vi "GetValueFromModelFile.vi"(8 "error in (no error)":errorcluster caption="에러 입력(에러 없음)", 11 "init 파일 경로":string) -> (3 "출력 클러스터":T1)   [LabVIEW 2018]
uses:
  <vilib>/Utility/config.llb/NI_LVConfig.lvlib
  <vilib>/Utility/config.llb/Read Key (String).vi
  ModelFileData.ctl
  <vilib>/Utility/config.llb/Read Key (Double).vi
  <vilib>/Utility/config.llb/Read Key (U32).vi
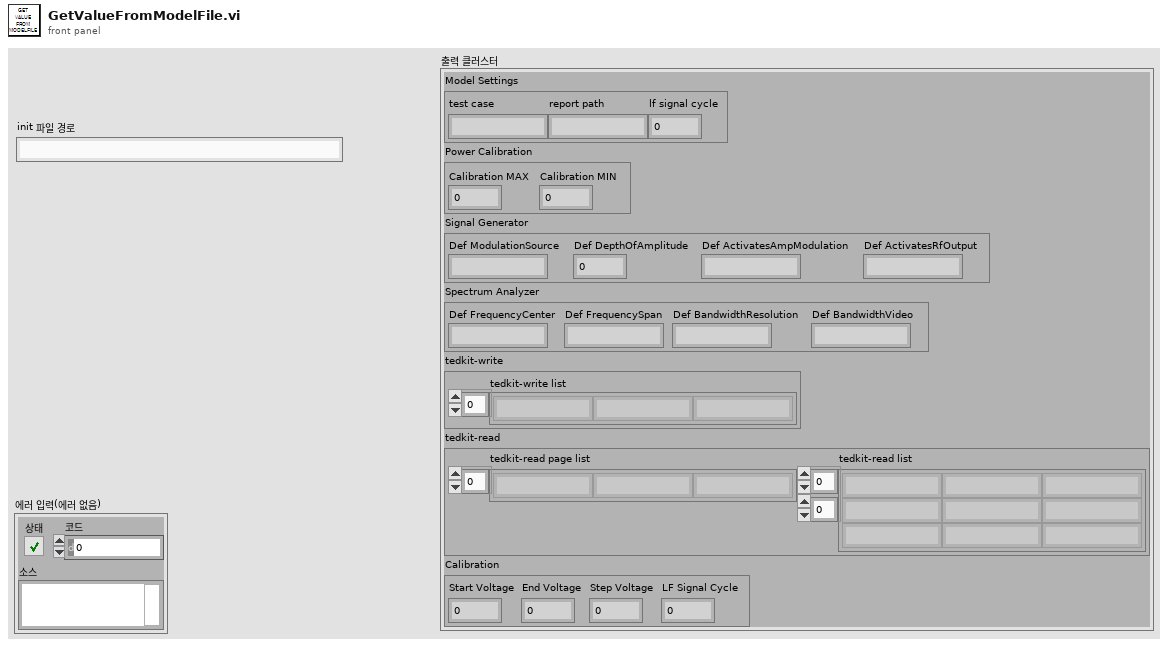
[diagram p1: front panel]
types:
  T1 = typedef "ModelFileData.ctl" = cluster{"Model Settings":cluster{"test case":string, "report path":string, "lf signal cycle":u16}, "Power Calibration":cluster{"Calibration MAX":dbl, "Calibration MIN":dbl}, "Signal Generator":cluster{"Def ModulationSource":string, "Def DepthOfAmplitude":dbl, "Def ActivatesAmpModulation":string, "Def ActivatesRfOutput":string}, "Spectrum Analyzer":cluster{"Def FrequencyCenter":string, "Def FrequencySpan":string, "Def BandwidthResolution":string, "Def BandwidthVideo":string}, "tedkit-write":cluster{"tedkit-write list":string[]}, "tedkit-read":cluster{"tedkit-read page list":string[], "tedkit-read list":string[][]}, "Calibration":cluster{"Start Voltage":dbl, "End Voltage":dbl, "Step Voltage":dbl, "LF Signal Cycle":u16}}
  T2 = typedef "NI_LVConfig.lvlib/Config Data RefNum.ctl" = refnum<k1>
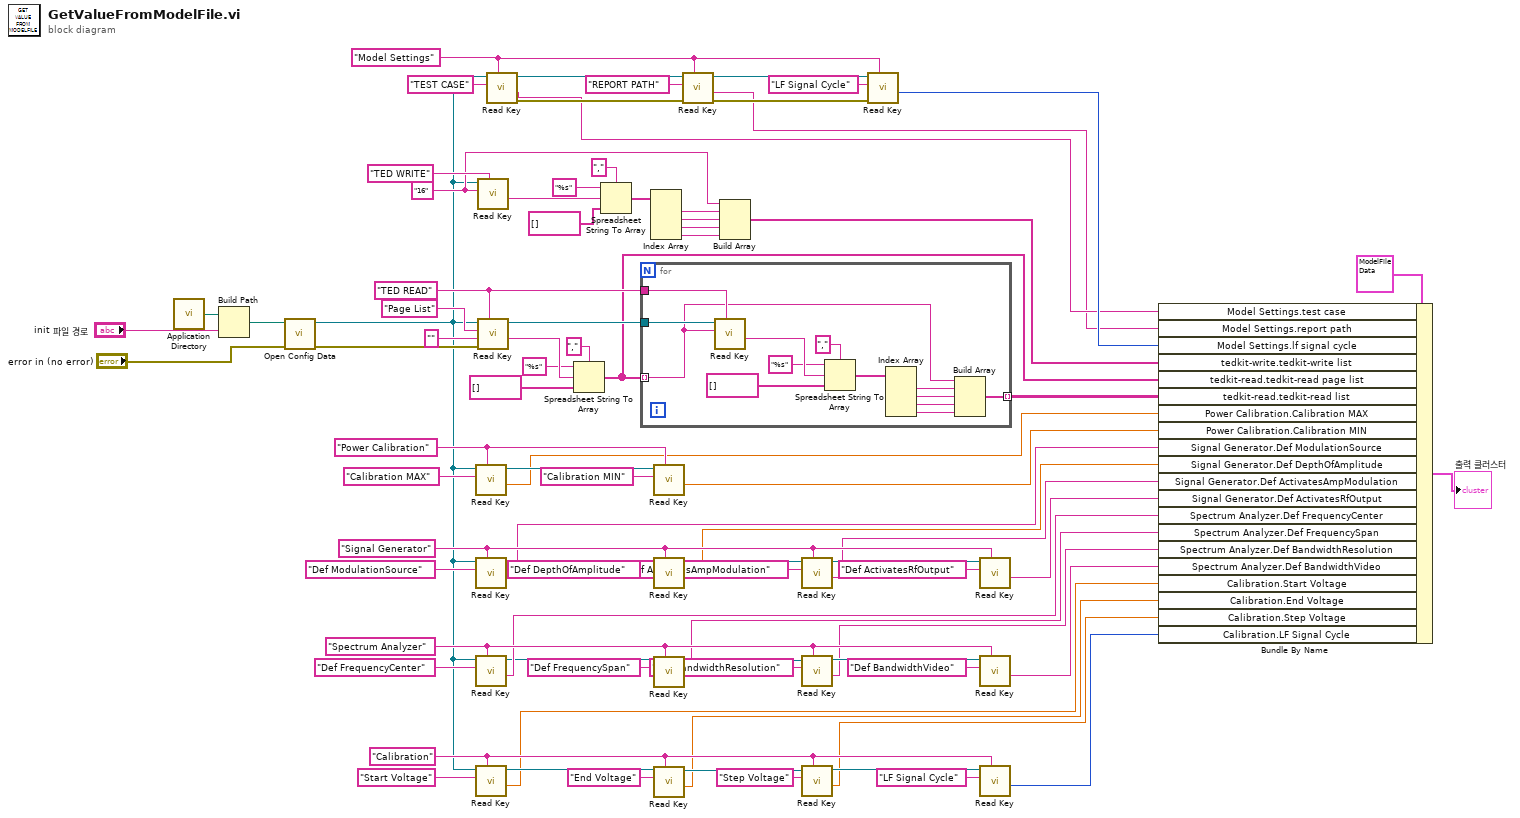
[diagram p0: block diagram]
diagram:
  w5 = "Model Settings" ("section")
  w22 = "Calibration" ("section")
  w33 = "Spectrum Analyzer" ("section")
  w46 = "Signal Generator" ("section")
  w25 = "16" ("key")
  w69 = "Power Calibration" ("section")
  w71 = "TED READ" ("section")
  n1 = call <vilib>:"Application Directory.vi"() -> ("Application Directory"=w83:path)
  n2 = Build Path(base path=w83, name or relative path="init 파일 경로") -> (appended path=w82:path)
  n3 = call <vilib>:"Open Config Data.vi"("error in (no error)"="error in (no error)", "configuration file path"=w82) -> ("error out"=w77:errorcluster, "refnum"=w12:T2)  [unwired: 7 in, 1 out]
  n4 = call-poly <vilib>:"Read Key.vi"("section"=w69, "key"="Calibration MAX", "refnum"=w12) -> ("value"=w63:dbl, "refnum out"=w70:T2)  [unwired: 5 in, 2 out]
  n5 = call-poly <vilib>:"Read Key.vi"("section"=w46, "key"="Def ModulationSource", "refnum"=w12) -> ("value"=w45:string, "refnum out"=w43:T2)  [unwired: 5 in, 2 out]
  n6 = call-poly <vilib>:"Read Key.vi"("section"=w33, "key"="Def FrequencyCenter", "refnum"=w12) -> ("value"=w32:string, "refnum out"=w27:T2)  [unwired: 5 in, 2 out]
  n7 = call-poly <vilib>:"Read Key.vi"("section"=w22, "key"="Start Voltage", "refnum"=w12) -> ("value"=w16:dbl, "refnum out"=w23:T2)  [unwired: 5 in, 2 out]
  n8 = call-poly <vilib>:"Read Key.vi"("section"="TED WRITE", "key"=w25, "refnum"=w12) -> ("value"=w59:string)  [unwired: 5 in, 3 out]
  n9 = call-poly <vilib>:"Read Key.vi"("section"=w71, "error in (no error)"=w77, "default value"="", "key"="Page List", "refnum"=w12) -> ("value"=w76:string, "refnum out"=w72:T2)  [unwired: 3 in, 2 out]
  n10 = call-poly <vilib>:"Read Key.vi"("section"=w5, "key"="TEST CASE", "refnum"=w12) -> ("error out"=w10:errorcluster, "value"=w2:string, "refnum out"=w9:T2)  [unwired: 5 in, 1 out]
  n11 = Spreadsheet String To Array(delimiter (Tab)="," ("구분 문자 (탭)"), format string="%s" ("포맷 문자열"), spreadsheet string=w76, array type (2D Dbl)=string[] [] ("배열 타입(2D Dbl)")) -> (array=w65:string[])
  n12 = Spreadsheet String To Array(delimiter (Tab)="," ("구분 문자 (탭)"), format string="%s" ("포맷 문자열"), spreadsheet string=w59, array type (2D Dbl)=string[] [] ("배열 타입(2D Dbl)")) -> (array=w57:string[])
  n13 = for {
    tunnel: w72 -> [w95]
    tunnel: w65 -> [w89] mode=indexing
    tunnel: w71 -> [w96]
    tunnel: [w84] -> w64 mode=indexing
    n14 = call-poly <vilib>:"Read Key.vi"("section"=w96, "key"=w89, "refnum"=w95) -> ("value"=w92:string)  [unwired: 5 in, 3 out]
    n15 = Spreadsheet String To Array(delimiter (Tab)="," ("구분 문자 (탭)"), format string="%s" ("포맷 문자열"), spreadsheet string=w92, array type (2D Dbl)=string[] [] ("배열 타입(2D Dbl)")) -> (array=w90:string[])
    n16 = Index Array(array=w90) -> (element #1=w88:string, element #2=w87:string, element #3=w86:string, element #4=w85:string)  [unwired: 4 in]
    n17 = Build Array(w89, w88, w87, w86, w85) -> (w84:string[])
  }
  n18 = Index Array(array=w57) -> (element #1=w56:string, element #2=w55:string, element #3=w54:string, element #4=w53:string)  [unwired: 4 in]
  n19 = call-poly <vilib>:"Read Key.vi"("section"=w69, "key"="Calibration MIN", "refnum"=w70) -> ("value"=w62:dbl)  [unwired: 5 in, 3 out]
  n20 = call-poly <vilib>:"Read Key.vi"("section"=w46, "key"="Def DepthOfAmplitude", "refnum"=w43) -> ("value"=w44:dbl, "refnum out"=w42:T2)  [unwired: 5 in, 2 out]
  n21 = call-poly <vilib>:"Read Key.vi"("section"=w33, "key"="Def FrequencySpan", "refnum"=w27) -> ("value"=w31:string, "refnum out"=w26:T2)  [unwired: 5 in, 2 out]
  n22 = call-poly <vilib>:"Read Key.vi"("section"=w22, "key"="End Voltage", "refnum"=w23) -> ("value"=w15:dbl, "refnum out"=w24:T2)  [unwired: 5 in, 2 out]
  n23 = call-poly <vilib>:"Read Key.vi"("section"=w5, "error in (no error)"=w10, "key"="REPORT PATH", "refnum"=w9) -> ("error out"=w7:errorcluster, "value"=w1:string, "refnum out"=w6:T2)  [unwired: 4 in, 1 out]
  n24 = Build Array(w25, w56, w55, w54, w53) -> (w51:string[])
  n25 = call-poly <vilib>:"Read Key.vi"("section"=w46, "key"="Def ActivatesAmpModulation", "refnum"=w42) -> ("value"=w40:string, "refnum out"=w41:T2)  [unwired: 5 in, 2 out]
  n26 = call-poly <vilib>:"Read Key.vi"("section"=w33, "key"="Def BandwidthResolution", "refnum"=w26) -> ("value"=w30:string, "refnum out"=w38:T2)  [unwired: 5 in, 2 out]
  n27 = call-poly <vilib>:"Read Key.vi"("section"=w22, "key"="Step Voltage", "refnum"=w24) -> ("value"=w14:dbl, "refnum out"=w17:T2)  [unwired: 5 in, 2 out]
  n28 = call-poly <vilib>:"Read Key.vi"("section"=w5, "error in (no error)"=w7, "key"="LF Signal Cycle", "refnum"=w6) -> ("value"=w3:u32)  [unwired: 4 in, 3 out]
  n29 = call-poly <vilib>:"Read Key.vi"("section"=w46, "key"="Def ActivatesRfOutput", "refnum"=w41) -> ("value"=w39:string)  [unwired: 5 in, 3 out]
  n30 = call-poly <vilib>:"Read Key.vi"("section"=w33, "key"="Def BandwidthVideo", "refnum"=w38) -> ("value"=w29:string)  [unwired: 5 in, 3 out]
  n31 = call-poly <vilib>:"Read Key.vi"("section"=w22, "key"="LF Signal Cycle", "refnum"=w17) -> ("value"=w13:u32)  [unwired: 5 in, 3 out]
  n32 = Bundle By Name(cluster=T1 {"Model Settings"={"test case"="", "report path"="", "lf signal cycle"=0}, "Power Calibration"={"Calibration MAX"=0.0, "Calibration MIN"=0.0}, "Signal Generator"={"Def ModulationSource"="", "Def DepthOfAmplitude"=0.0, "Def ActivatesAmpModulation"="", "Def ActivatesRfOutput"=""}, "Spectrum Analyzer"={"Def FrequencyCenter"="", "Def FrequencySpan"="", "Def BandwidthResolution"="", "Def BandwidthVideo"=""}, "tedkit-write"={"tedkit-write list"=[]}, "tedkit-read"={"tedkit-read page list"=[], "tedkit-read list"=[]}, "Calibration"={"Start Voltage"=0.0, "End Voltage"=0.0, "Step Voltage"=0.0, "LF Signal Cycle"=0}} ("ModeFileData"), "Model Settings.test case"=w2, "Model Settings.report path"=w1, "Model Settings.lf signal cycle"=w3, "tedkit-write.tedkit-write list"=w51, "tedkit-read.tedkit-read page list"=w65, "tedkit-read.tedkit-read list"=w64, "Power Calibration.Calibration MAX"=w63, "Power Calibration.Calibration MIN"=w62, "Signal Generator.Def ModulationSource"=w45, "Signal Generator.Def DepthOfAmplitude"=w44, "Signal Generator.Def ActivatesAmpModulation"=w40, "Signal Generator.Def ActivatesRfOutput"=w39, "Spectrum Analyzer.Def FrequencyCenter"=w32, "Spectrum Analyzer.Def FrequencySpan"=w31, "Spectrum Analyzer.Def BandwidthResolution"=w30, "Spectrum Analyzer.Def BandwidthVideo"=w29, "Calibration.Start Voltage"=w16, "Calibration.End Voltage"=w15, "Calibration.Step Voltage"=w14, "Calibration.LF Signal Cycle"=w13) -> (→"출력 클러스터":T1)
